vi "AlliGator Save Multiple ROIs v3.vi"(8 "Error In":errorcluster, 9 "Default File Name":string="Multiple ROIs.roiN", 10 "Destination Folder (Default: last)":path=path "", 11 "ROI Description":T1 {"Named ROI Descriptions"."ROI Descriptor"."Contours"."Type" items=["No Selection", "Point", "Line", "Rectangle", "Oval", "Polygon", "Freehand Region", "Annulus", "Unused2", "Unused3", "Broken Line", "Freehand Line", "Rotated Rectangle"]}) -> (0 "Error Out":errorcluster, 3 "Notebook Message":string)   [LabVIEW 2021, in "AlliGator ROIs.lvlib"]
doc: "Save multiple ROIs."
uses:
  Image/Image Control Multiple ROIs Description v2.ctl
  Image/Named ROI Description.ctl
  2f6536f2-4c73-4be5-9a90-4bb6a5b7d0f4.vi
  <vilib>/JDP Science/JSONtext/Variant to JSON Text.vi
  <vilib>/JDP Science/JSONtext/LVClass Serializer/JSONtext LVClass Serializer.lvclass
  AlliGator ROIs.lvlib
  Image/Image.lvlib
panel:
  # "see the AlliGator License on the block diagram (Ctrl+E or Window:Show Block Diagram)"
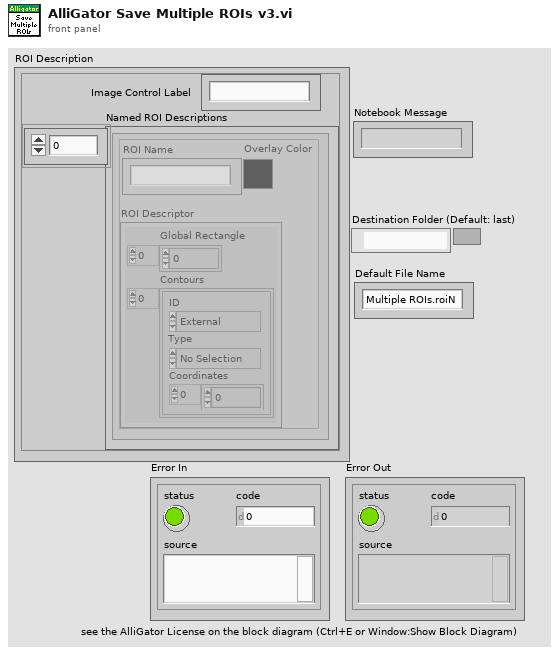
[diagram p1: front panel]
types:
  T1 = typedef "Image.lvlib/Image Control Multiple ROIs Description v2.ctl" = cluster{"Image Control Label":string, "Named ROI Descriptions":T2[]}
  T2 = typedef "Image.lvlib/Named ROI Description.ctl" = cluster{"ROI Descriptor":T3, "ROI Name":string, "Overlay Color":u32}
  T3 = typedef "ROI Descriptor" = cluster{"Global Rectangle":i32[], "Contours":cluster{"ID":enum32{"External", "Internal"}, "Type":u32, "Coordinates":i32[]}[]}
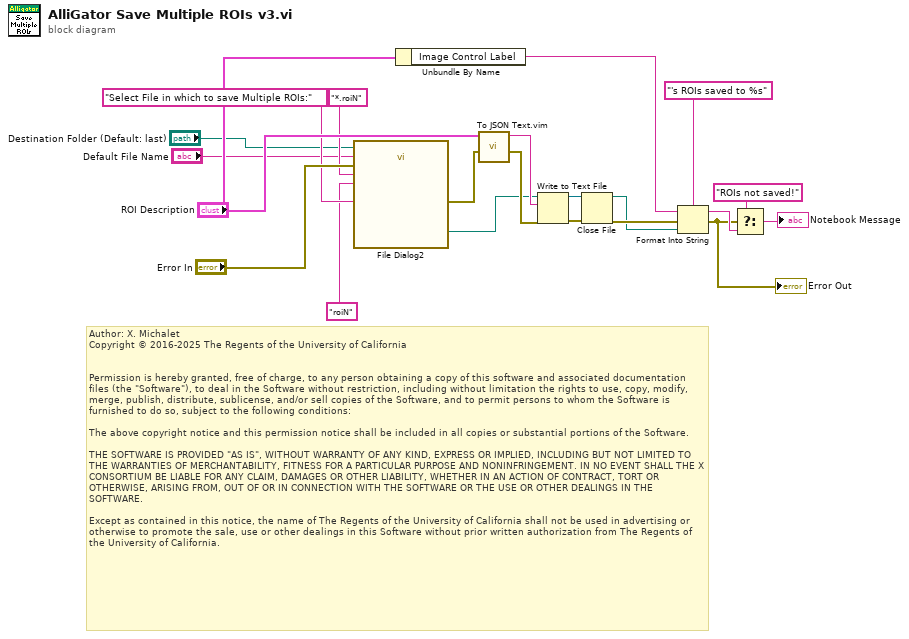
[diagram p0: block diagram]
diagram:
  # "Author: X. Michalet\nCopyright © 2016-2025 The Regents of the University of California\n \n\nPermission is hereby granted, free of charge, to any person obtaining a copy of this software and associated documentation files (the \"Software\"), to deal in the Software without restriction, including without limitation the rights to use, copy, modify, merge, publish, distribute, sublicense, and/or sell copies of the Software, and to permit persons to whom the Software is furnished to do so, subject to the following conditions:\n\nThe above copyright notice and this permission notice shall be included in all copies or substantial portions of the Software.\n\nTHE SOFTWARE IS PROVIDED \"AS IS\", WITHOUT WARRANTY OF ANY KIND, EXPRESS OR IMPLIED, INCLUDING BUT NOT LIMITED TO THE WARRANTIES OF MERCHANTABILITY, FITNESS FOR A PARTICULAR PURPOSE AND NONINFRINGEMENT. IN NO EVENT SHALL THE X CONSORTIUM BE LIABLE FOR ANY CLAIM, DAMAGES OR OTHER LIABILITY, WHETHER IN AN ACTION OF CONTRACT, TORT OR OTHERWISE, ARISING FROM, OUT OF OR IN CONNECTION WITH THE SOFTWARE OR THE USE OR OTHER DEALINGS IN THE SOFTWARE.\n\nExcept as contained in this notice, the name of The Regents of the University of California shall not be used in advertising or otherwise to promote the sale, use or other dealings in this Software without prior written authorization from The Regents of the University of California."
  n1 = call "File Dialog2"("start path"="Destination Folder (Default: last)", "prompt"="Select File in which to save Multiple ROIs:" ("Prompt"), "default name"="Default File Name", "error in"="Error In", "pattern (all files)"="*.roiN" ("Pattern (*.xml;*.XML)"), "pattern label"="roiN" ("File Extension (xml)")) -> ("selected path"=w2:path, "error out"=w3:errorcluster)  [unwired: 6 in, 2 out]
  n2 = Unbundle By Name("ROI Description") -> ("Image Control Label"=w15:string)
  n3 = call "To JSON Text.vim"("error in (no error)"=w3, "Anything"="ROI Description") -> ("error out"=w4:errorcluster, "<JSON>"=w6:string)  [unwired: 8 in]
  n4 = Write to Text File(file (use dialog)=w2, text=w6, error in=w4) -> (refnum out=w7:refnum<file>, error out=w5:errorcluster)  [unwired: 1 in, 1 out]
  n5 = Close File(refnum=w7, error in=w5) -> (path=w17:path, error out=w18:errorcluster)
  n6 = Format Into String(format string="'s ROIs saved to %s", initial string=w15, error in=w18, w17) -> (resulting string=w19:string, error out=w12:errorcluster)
  "Error Out" <- w12
  n7 = Select(t="ROIs not saved!", s=w12, f=w19) -> (s? t:f=→"Notebook Message":string)
